vi "SWERVE DRIVE one corner.vi"(0 "velocity in":dbl, 1 "steer angle in\n(deg)":dbl, 2 "distance (ft)":dbl, 3 "Control Mode":T1, 5 "error in (no error)":errorcluster, 6 "drive\nmotor":T9 {"gear ratio" format="%_5f"; "MOTOR SELECT" items=["REV NEO"=5676, "REV NEO 550"=11000, "VEX Falcon"=6380, "WC Kraken"=6000]}, 7 "swerve module in":T2 {"corner wt (lbm)" format="%_4f"; "POS" format="%.3g"; "coord wrt geom CTR"."Y" format="%.4g"; "coord wrt geom CTR"."X" format="%.4g"; "from pivot to module"."theta park (deg)" format="%.4g"; "from pivot to module"."theta spin (deg)" format="%.4g"; "from pivot to module"."theta (deg)" format="%.4g"; "from pivot to module"."R" format="%.4g"; "ABS" format="%.3g"; "target" format="%.3g"; "V" format="%.3g"}, 8 "steering\nmotor":T9 {"gear ratio" format="%_5f"; "MOTOR SELECT" items=["REV NEO"=5676, "REV NEO 550"=11000, "VEX Falcon"=6380, "WC Kraken"=6000]}, 9 "DeviceRefs":cluster{"Driver":T3, "Steer":T3, "Encoder":T8}) -> (13 "swerve module out":T2 {"corner wt (lbm)" format="%_4f"; "POS" format="%.3g"; "coord wrt geom CTR"."Y" format="%.4g"; "coord wrt geom CTR"."X" format="%.4g"; "from pivot to module"."theta park (deg)" format="%.4g"; "from pivot to module"."theta spin (deg)" format="%.4g"; "from pivot to module"."theta (deg)" format="%.4g"; "from pivot to module"."R" format="%.4g"; "ABS" format="%.3g"; "target" format="%.3g"; "V" format="%.3g"}, 14 "velocity out":dbl, 15 "steer angle out\n(deg)":dbl, 19 "error out":errorcluster)   [LabVIEW 2023]
uses:
  ctrl defs/ctrl swerve motor.ctl
  ctrl defs/ctrl MOTOR SELECT.ctl
  <vilib>/Rock Robotics/WPI/ThirdParty/REV Robotics/REVLib/Typedef/Spark MAX Idle Mode.ctl
  ctrl defs/ctrl Spark MAX current limiting.ctl
  ctrl defs/ctrl motor PIDF coefficients.ctl
  <vilib>/Rock Robotics/WPI/ThirdParty/REV Robotics/REVLib/Typedef/Spark MAX Smart Motion Parameters.ctl
  <vilib>/Rock Robotics/WPI/MotorControl/WPI_MotorControlDeviceRef.ctl
  <vilib>/Rock Robotics/WPI/MotorControl/WPI_MotorControlType.ctl
  <vilib>/Rock Robotics/SystemInterfaces/DIO/FPGA_DIOPWMChannel.ctl
  <vilib>/Rock Robotics/WPI/PWM/WPI_PWMDeadband.ctl
  <vilib>/Rock Robotics/SystemInterfaces/DIO/FPGA_DIOChannel.ctl
  <vilib>/Rock Robotics/WPI/ThirdParty/Phoenix-LabVIEW/CANCoder/Controls/CTRE_Phoenix_CANcoder_DeviceRef.ctl
  ctrl defs/ctrl swerve module.ctl
  <vilib>/Rock Robotics/WPI/ThirdParty/REV Robotics/REVLib/Typedef/Spark MAX Control Type.ctl
  <vilib>/Rock Robotics/WPI/ThirdParty/Phoenix-LabVIEW/CANCoder/Get/CTRE_Phoenix_CANcoder_GetSensorData.vi
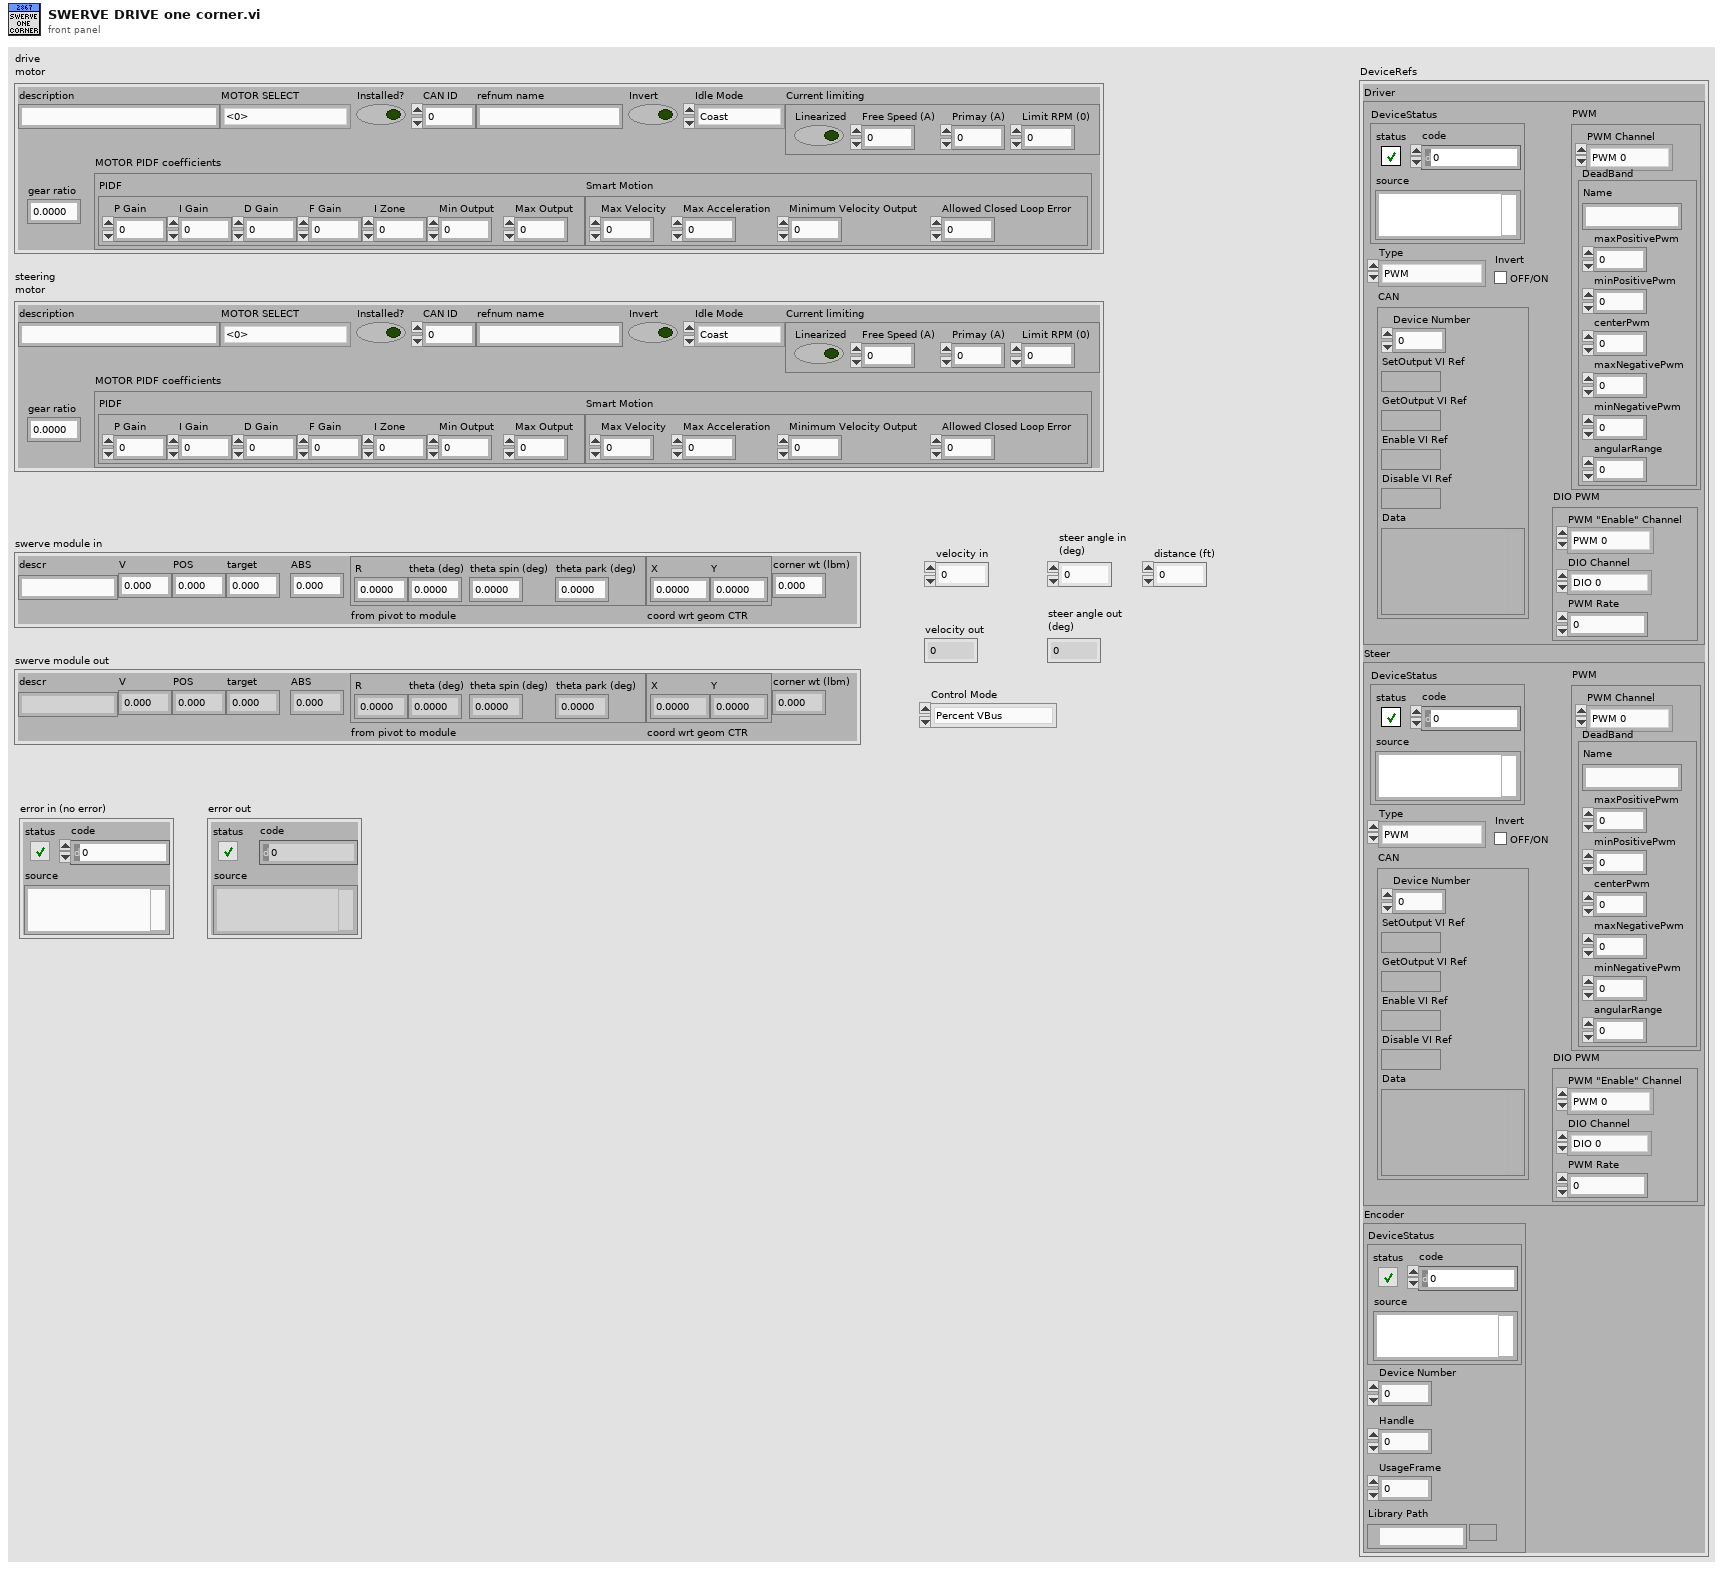
[diagram p1: front panel]
types:
  T1 = typedef "Spark MAX Control Type.ctl" = enum16{"Percent VBus", "Voltage", "Velocity", "Position", "Smart Motion", "Current", "Smart Velocity"}
  T2 = typedef "ctrl swerve module.ctl" = cluster{"descr":string, "V":dbl, "POS":dbl, "target":dbl, "ABS":dbl, "from pivot to module":cluster{"R":dbl, "theta (deg)":dbl, "theta spin (deg)":dbl, "theta park (deg)":dbl}, "coord wrt geom CTR":cluster{"X":dbl, "Y":dbl}, "corner wt (lbm)":dbl}
  T3 = typedef "WPI_MotorControlDeviceRef.ctl" = cluster{"DeviceStatus":errorcluster, "Type":T4, "PWM":cluster{"PWM Channel":T5, "DeadBand":T6}, "CAN":cluster{"Device Number":u8, "SetOutput VI Ref":variant, "GetOutput VI Ref":variant, "Enable VI Ref":variant, "Disable VI Ref":variant, "Data":variant}, "Invert":bool, "DIO PWM":cluster{"PWM \"Enable\" Channel":T5, "DIOChannel":T7, "PWM Rate":dbl}}
  T4 = typedef "WPI_MotorControlType.ctl" = enum16{"PWM", "CAN", "DIO PWM"}
  T5 = typedef "FPGA_DIOPWMChannel.ctl" = enum8{"PWM 0", "PWM 1", "PWM 2", "PWM 3", "PWM 4", "PWM 5", "PWM 6", "PWM 7", "PWM 8", "PWM 9", "PWM MXP 0", "PWM MXP 1", "PWM MXP 2", "PWM MXP 3", "PWM MXP 4", "PWM MXP 5", "PWM MXP 6", "PWM MXP 7", "PWM MXP 8", "PWM MXP 9", "Invalid"}
  T6 = typedef "WPI_PWMDeadband.ctl" = cluster{"Name":string, "maxPositivePwm":i32, "minPositivePwm":i32, "centerPwm":i32, "maxNegativePwm":i32, "minNegativePwm":i32, "angularRange":u16}
  T7 = typedef "FPGA_DIOChannel.ctl" = enum8{"DIO 0", "DIO 1", "DIO 2", "DIO 3", "DIO 4", "DIO 5", "DIO 6", "DIO 7", "DIO 8", "DIO 9", "DIO MXP 0", "DIO MXP 1", "DIO MXP 2", "DIO MXP 3", "DIO MXP 4", "DIO MXP 5", "DIO MXP 6", "DIO MXP 7", "DIO MXP 8", "DIO MXP 9", "DIO MXP 10", "DIO MXP 11", "DIO MXP 12", "DIO MXP 13", "DIO MXP 14", "DIO MXP 15", "SPI Port CS1", "SPI Port CS2", "SPI Port CS3", "SPI Port MISO", "SPI Port MOSI", "Invalid"}
  T8 = typedef "CTRE_Phoenix_CANcoder_DeviceRef.ctl" = cluster{"DeviceStatus":errorcluster, "Device Number":u8, "Handle":u64, "UsageFrame":u32, "Library Path":path}
  T9 = typedef "ctrl swerve motor.ctl" = cluster{"description":string, "MOTOR SELECT":T10, "Installed?":bool, "CAN ID":u8, "refnum name":string, "Invert":bool, "Idle Mode":T11, "Current limiting":T12, "MOTOR PIDF coefficients":T13, "gear ratio":dbl}
  T10 = typedef "ctrl MOTOR SELECT.ctl" = i16
  T11 = typedef "Spark MAX Idle Mode.ctl" = enum16{"Coast", "Brake"}
  T12 = typedef "ctrl Spark MAX current limiting.ctl" = cluster{"Linearized":bool, "Free Speed (A)":dbl, "Primay (A)":dbl, "Limit RPM (0)":u32}
  T13 = typedef "ctrl motor PIDF coefficients.ctl" = cluster{"PIDF":cluster{"P Gain":dbl, "I Gain":dbl, "D Gain":dbl, "F Gain":dbl, "I Zone":dbl, "Min Output":dbl, "Max Output":dbl}, "Smart Motion":T14}
  T14 = typedef "Spark MAX Smart Motion Parameters.ctl" = cluster{"Max Velocity":dbl, "Max Acceleration":dbl, "Minimum Velocity Output":dbl, "Allowed Closed Loop Error":dbl}
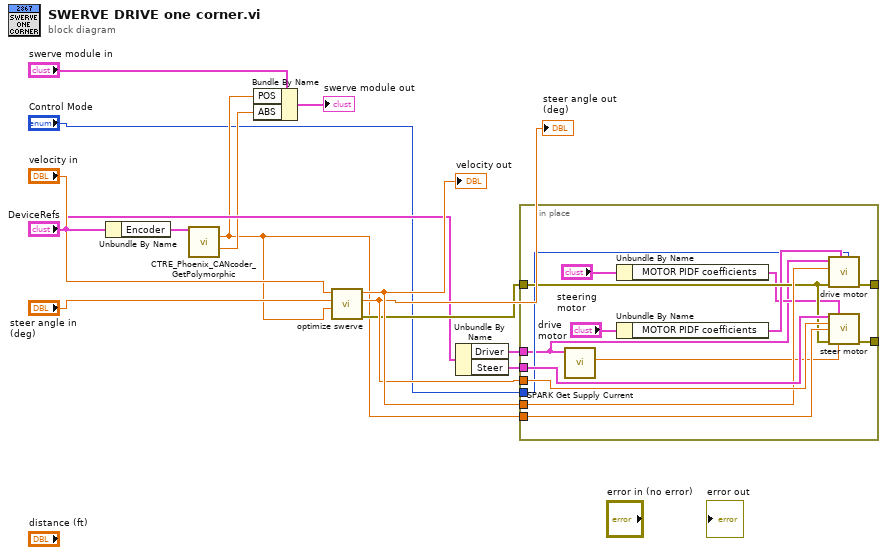
[diagram p0: block diagram]
diagram:
  n1 = Unbundle By Name("DeviceRefs") -> ("Encoder"=w14:T8)
  n2 = call-poly <vilib>:"CTRE_Phoenix_CANcoder_GetPolymorphic.vi"("CTRE_CANcoder_DeviceRef"=w14) -> ("Position"=w5:dbl, "Absolute Position"=w6:dbl)  [unwired: 10 in, 3 out]
  n3 = Bundle By Name(cluster="swerve module in", "POS"=w5, "ABS"=w6) -> (→"swerve module out":T2)
  n4 = call "optimize swerve.vi"("current angle (deg)"=w5, "target angle (deg)"="steer angle in\n(deg)", "velocity"="velocity in") -> ("error out"=w9:errorcluster, "steer angle (deg)"=w12:dbl, "velocity"=w13:dbl)  [unwired: 5 in, 1 out]
  "velocity out" <- w13
  "steer angle out\n(deg)" <- w12
  n5 = Unbundle By Name("DeviceRefs") -> ("Driver"=w7:T3, "Steer"=w2:T3)
  n6 = in-place {
    in-place-border: w12 -> [w28]
    in-place-border: w2 -> [w27]
    in-place-border: w5 -> [w26]
    in-place-border: w7 -> [w16]
    in-place-border: w13 -> [w25]
    in-place-border: w9 -> [w24]
    in-place-border: [w23] -> _
    in-place-border: [w22] -> _
    in-place-border: "Control Mode" -> [w17]
    n7 = call <vilib>:"SPARK Get Supply Current.vi"("MotorControlDevRef in"=w16) -> ("Current"=w15:dbl)  [unwired: 7 in, 3 out]
    n8 = Unbundle By Name("steering\nmotor") -> ("MOTOR PIDF coefficients"=w19:T13)
    n9 = Unbundle By Name("drive\nmotor") -> ("MOTOR PIDF coefficients"=w21:T13)
    n10 = call "drive motor.vi"("Control Mode"=w17, "MOTOR PIDF coefficients"=w21, "error in (no error)"=w24, "velocity"=w25, "Driver"=w16) -> ("error out"=w23:errorcluster)  [unwired: 6 in]
    n11 = call "steer motor.vi"("MotorControlDevRef"=w27, "MOTOR PIDF coefficients"=w19, "target"=w28, "encoder"=w26, "error in (no error)"=w24, "DRIVE motor\ncurrent (A)"=w15) -> ("error out"=w22:errorcluster)  [unwired: 9 in]
  }
